vi "Exercises_7-1-1.vi"(8 "error in (no error)":errorcluster, 9 "Min Temp":dbl, 10 "Max Temp":dbl, 11 "Current Temp":dbl) -> (0 "error out":errorcluster, 1 "Warning?":bool, 2 "Warning Text":string)   [LabVIEW 2014]
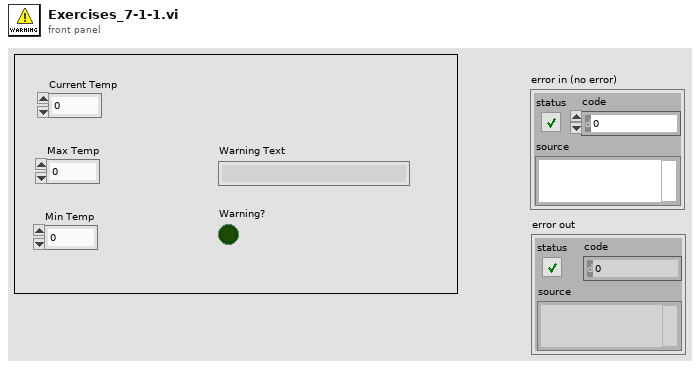
[diagram p1: front panel]
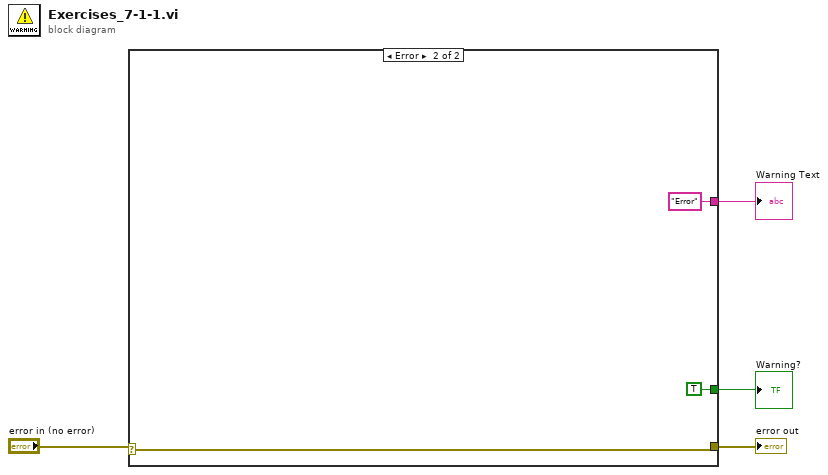
[diagram p0: block diagram]
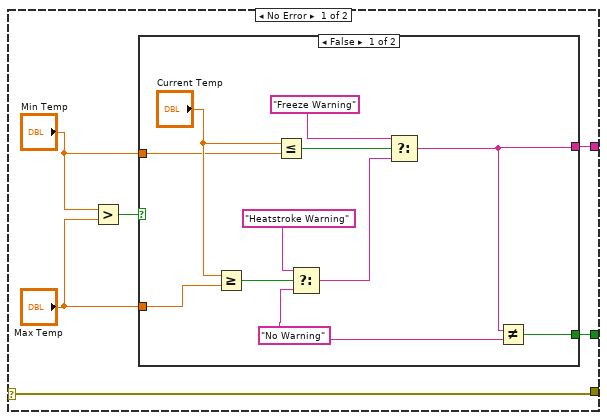
[diagram p2: hidden frame]
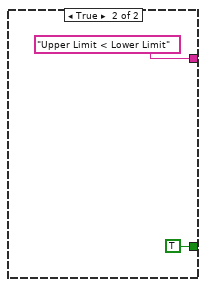
[diagram p3: hidden frame]
diagram:
  n1 = case shown="Error" "error in (no error)" {
    selector: "error in (no error)" -> [w5 w26]
    tunnel: [w10 "Error"] -> w4
    tunnel: [w9 TRUE] -> w3
    tunnel: [w5 w26] -> w2
    frame No Error {
      n2 = Greater?(x="Min Temp", y="Max Temp") -> (0:w6:bool)
      n3 = case shown="False" w6 {
        tunnel: [w15 "Upper Limit < Lower Limit"] -> w10
        tunnel: [w13 TRUE] -> w9
        tunnel: "Min Temp" -> [w12 _]
        tunnel: "Max Temp" -> [w11 _]
        frame False {
          w14 = "No Warning"
          n4 = Greater Or Equal?(x="Current Temp", y=w11) -> (x >= y?=w21:bool)
          n5 = Less Or Equal?(x="Current Temp", y=w12) -> (x <= y?=w18:bool)
          n6 = Select(t="Heatstroke Warning", s=w21, f=w14) -> (s? t:f=w17:string)
          n7 = Select(t="Freeze Warning", s=w18, f=w17) -> (s? t:f=w15:string)
          n8 = Not Equal?(x=w15, y=w14) -> (x != y?=w13:bool)
        }
        frame True {
        }
      }
    }
    frame Error {
    }
  }
  "Warning Text" <- w4
  "Warning?" <- w3
  "error out" <- w2
